vi "U6 easy Stream Full.vi"() -> ()   [LabVIEW 2021]
panel:
  in  "Simulated Processing Delay [ms]":u32
  in  "Iterations/Second":i32=1
  in  "Binary":bool
  in  "StreamSettlingFactor":i32
  in  "Resolution Index":u8
  in  "Range Constants":u8[](array[ring])=[0, 0, 0, 0] items=["LJ_rgBIP10V", "LJ_rgBIP1V", "LJ_rgBIPP1V", "LJ_rgBIPP01V"]
  out "Stream Parameters":T1 {"Device Backlog [%]" format="%.2f"}
  in  "PC buffer size (seconds)":dbl=10.0 format="%.2f"
  in  "Scan List (-)":u8[](array[numeric])=[199, 199, 199, 199]
  out "Data":dbl[][](array[numeric]) format="%.3f"
  out "Waveform Graph":dbl[][](graph)
  in  "Scan List (+)":u8[](array[numeric])=[0, 1, 2, 3]
  out "# of iterations":i32
  in  "Scan Rate (Hz)":dbl=1000.0 format="%.3f"
  in  "stop":bool
  out "Error Message":string
  # "This example streams from the first found USB U6."
  # "The + scan list is the positive\nchannels.  For each element in\nthe + list, there must also be\nan element in the - list, which is\nthe negative channels.  For\nsingle-ended channels, put in\n199 for the negative channel.\n\nTo remove an element, right-click\non it, select Data Operations =>\nRemove Element.\n\nTo empty an array, right-click\nnear the edge, select Data\nOperations => Empty Array.\n\nOther useful operations:  From the\nOperate menu are \"Make Current\nValues Default\" and \"Reinitialize\nTo Default\"."
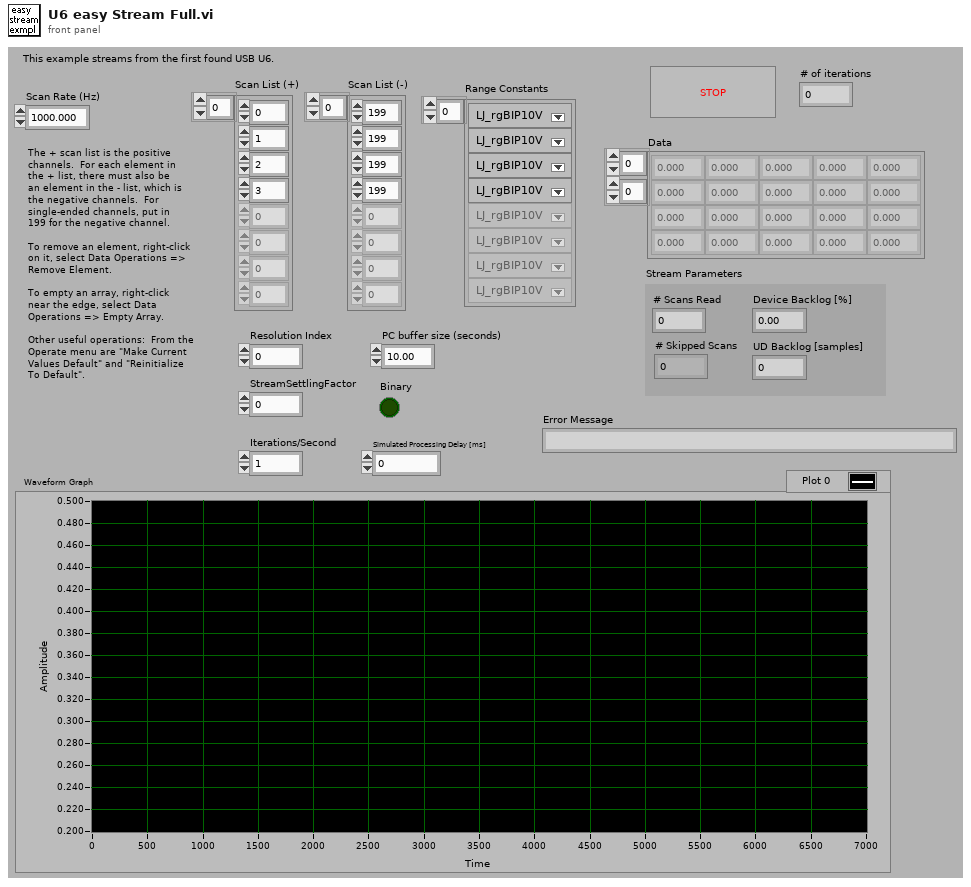
[diagram p1: front panel]
types:
  T1 = cluster{"# Scans Read":i32, "# Skipped Scans":i32, "Device Backlog [%]":dbl, "UD Backlog [samples]":i32}
  T2 = cluster{"PC buffer size (seconds)":dbl, "Resolution Index":u8, "StreamSettlingFactor":i32, "Binary":bool}
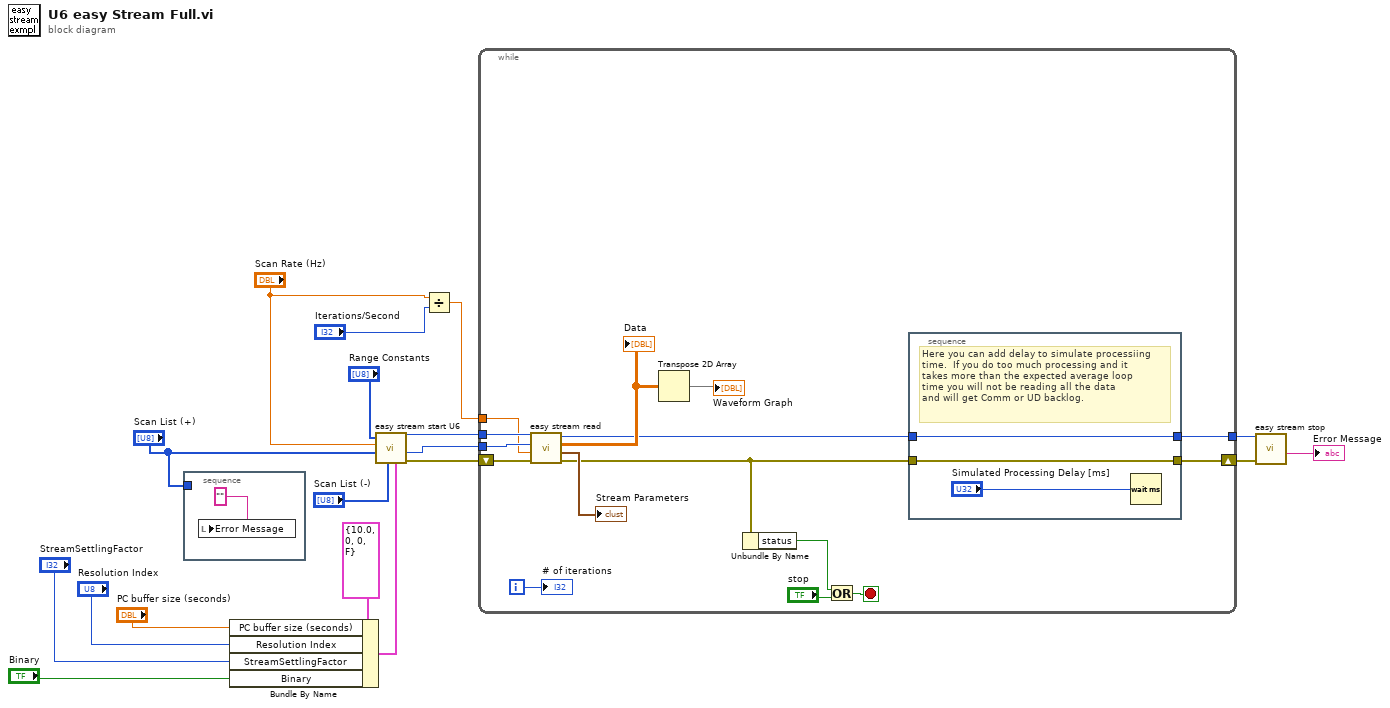
[diagram p0: block diagram]
diagram:
  n1 = stacked-sequence {
    tunnel: "Scan List (+)" -> [_]
    frame #0 {
      n2 = local write "Error Message"("" ("Error Message")) -> ()
    }
  }
  n3 = Bundle By Name(cluster=T2 {"PC buffer size (seconds)"=10.0, "Resolution Index"=0, "StreamSettlingFactor"=0, "Binary"=FALSE} ("Advanced"), "PC buffer size (seconds)"="PC buffer size (seconds)", "Resolution Index"="Resolution Index", "StreamSettlingFactor"="StreamSettlingFactor", "Binary"="Binary") -> (w8:T2)
  n4 = call "easy stream start U6.vi"("Advanced"=w8, "Scan List (-)"="Scan List (-)", "Scan List (+)"="Scan List (+)", "Scan Rate (Hz)"="Scan Rate (Hz)", "Range Constants"="Range Constants") -> ("error out"=w18:errorcluster, "# Channels"=w17:i32, "Handle Out"=w16:i32)  [unwired: 3 in, 1 out]
  n5 = Divide(x="Scan Rate (Hz)", y="Iterations/Second") -> (x/y=w1:dbl)
  n6 = while {
    tunnel: [w20] -> w14
    tunnel: w16 -> [w27]
    tunnel: w17 -> [w28]
    shift-left: w18 -> [w29]
    shift-right: [w21] -> w15
    tunnel: w1 -> [w24]
    i -> [w31]
    stop <- w32 stop-if-true
    n7 = call "easy stream read.vi"("error in"=w29, "Scans To Read"=w24, "# Channels In Stream"=w28, "Handle In"=w27) -> ("error out"=w23:errorcluster, "Stream Parameters"=→"Stream Parameters":T1, "Data"=w26:dbl[][], "Handle Out"=w22:i32)  [unwired: 4 in]
    "Data" <- w26
    n8 = Transpose 2D Array(2D array=w26) -> (transposed array=→"Waveform Graph":dbl[][])
    n9 = Unbundle By Name(w23) -> ("status"=w33:bool)
    n10 = Or(x=w33, y="stop") -> (x .or. y?=w32:bool)
    n11 = stacked-sequence {
      tunnel: w23 -> [w37]
      tunnel: [w37] -> w21
      tunnel: w22 -> [w36]
      tunnel: [w36] -> w20
      frame #0 {
        # "Here you can add delay to simulate processiing\ntime.  If you do too much processing and it\ntakes more than the expected average loop\ntime you will not be reading all the data\nand will get Comm or UD backlog."
        n12 = Wait (ms)(milliseconds to wait="Simulated Processing Delay [ms]") -> ()  [unwired: 1 out]
      }
    }
    "# of iterations" <- w31
  }
  n13 = call "easy stream stop.vi"("error in"=w15, "Handle In"=w14) -> ("Error Message"=→"Error Message":string)  [unwired: 7 in, 2 out]
